vi "ErrorCatcher.vi"(8 "error in (no error)":errorcluster, 10 "Test Daten":T1={"commandlist"="", "line"=0, "last response"="", "timeout"=0, "wait"=0, "erfolgreich"=FALSE, "next state"=enum."init", "Zustand"=enum."starting", "manual Test"=FALSE}, 11 "DeviceInterface in":refnum<class "DeviceInterface.lvclass">) -> (0 "error out":errorcluster, 3 "DeviceInterface out":refnum<class "DeviceInterface.lvclass">)   [LabVIEW 2013, in "DeviceInterface.lvclass"]
uses:
  DeviceInterface.lvclass
  Main/controls/TestData.ctl
  Main/controls/TestStates.ctl
  Main/controls/generalTestStates.ctl
  lib/EMV-Test.lvlib
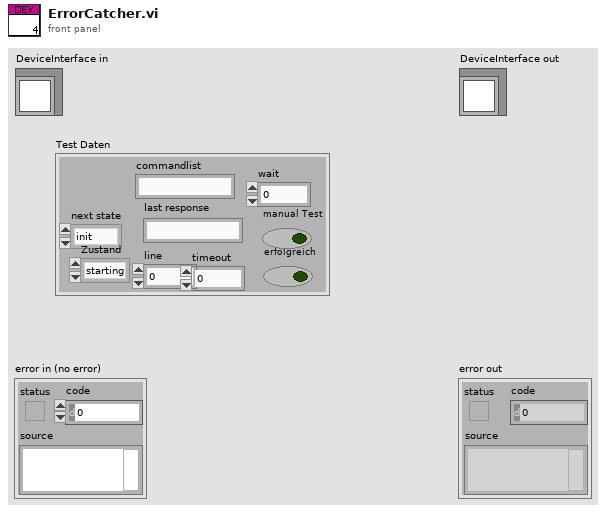
[diagram p1: front panel]
types:
  T1 = typedef "EMV-Test.lvlib/TestData.ctl" = cluster{"commandlist":string, "line":i32, "last response":string, "timeout":i32, "wait":u32, "erfolgreich":bool, "next state":T2, "Zustand":T3, "manual Test":bool}
  T2 = typedef "EMV-Test.lvlib/TestStates.ctl" = enum16{"event loop", "save Test", "Custom Action 1", "Custom Action 2", "pause", "vorgefertigter Test", "manueller Test", "respond to response", "error", "init", "start Test", "evaluate line", "wait for Response", "wait", "catch error", "close Connection", "end"}
  T3 = typedef "generalTestStates.ctl" = enum16{"paused", "starting", "waiting", "running", "finished"}
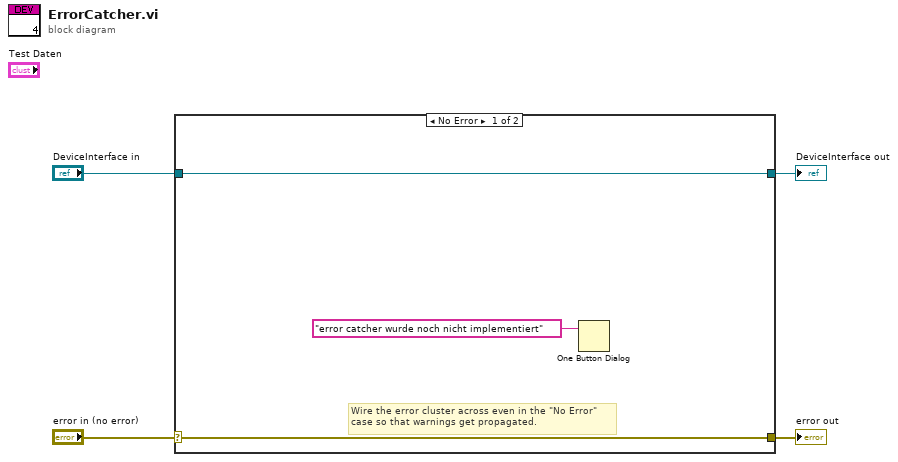
[diagram p0: block diagram]
diagram:
  n1 = case shown="No Error" "error in (no error)" {
    selector: "error in (no error)" -> [w6 w9]
    tunnel: [w6 w9] -> w3
    tunnel: [w7 w8] -> w1
    tunnel: "DeviceInterface in" -> [w7 w8]
    frame No Error {
      # "Wire the error cluster across even in the \"No Error\"\ncase so that warnings get propagated."
      n2 = One Button Dialog(message="error catcher wurde noch nicht implementiert") -> ()  [unwired: 1 in, 1 out]
    }
    frame Error {
    }
  }
  "error out" <- w3
  "DeviceInterface out" <- w1
